vi "Generate Trajectory.vi"(8 "Conditions":T2, 9 "Limits":T1={"Velocity (fps)"=6.0, "Acceleration (fps^2)"=15.0, "Jerk (fps^3)"=100.0}, 10 "WayPoints":cluster{"x":dbl, "y":dbl, "th":dbl}[](array[cluster]), 11 "Sample Period (s)":dbl=0.02) -> (0 "Updated Waypoints":cluster{"x":dbl, "y":dbl, "th":dbl}[](array[cluster]), 1 "Valid":bool, 2 "Time (s)":dbl, 3 "Trajectory Data":T3(array[cluster]), 4 "Distance (ft)":dbl)   [LabVIEW 2018]
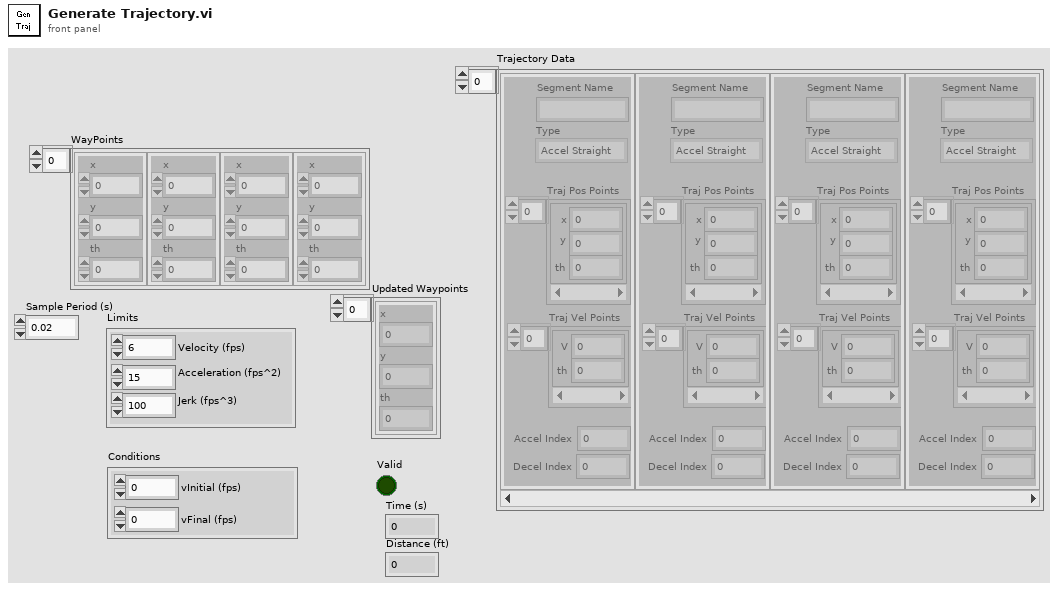
[diagram p1: front panel]
types:
  T1 = cluster{"Velocity (fps)":dbl, "Acceleration (fps^2)":dbl, "Jerk (fps^3)":dbl}
  T2 = cluster{"vInitial (fps)":dbl, "vFinal (fps)":dbl}
  T3 = cluster{"Segment Name":string, "Type":enum16{"Accel Straight", "Const Straight", "Blend", "Circle"}, "Traj Pos Points":cluster{"x":dbl, "y":dbl, "th":dbl}[], "Traj Vel Points":cluster{"V":dbl, "th":dbl}[], "Accel Index":i32, "Decel Index":i32}[]
  T4 = cluster{"distance (ft)":dbl, "dist of baseline Jerk":dbl, "dist of high Jerk":dbl}
  T5 = cluster{"Velocity (fps)":dbl, "Acceleration (fps^2)":dbl, "vInitial (fps)":dbl, "Sample Period (s)":dbl, "Jerk (fps^3)":dbl, cluster{"distance (ft)":dbl, "dist of baseline Jerk":dbl, "dist of high Jerk":dbl}, cluster{"distance (ft)":dbl, "dist of baseline Jerk":dbl, "dist of high Jerk":dbl}}
  T6 = cluster{"Point Out":cluster{"x":dbl, "y":dbl, "th":dbl}, "Point Out":cluster{"x":dbl, "y":dbl, "th":dbl}, "Valid":bool}[]
  T7 = typedef "BlendType.ctl" = cluster{"Scaling":dbl, "Length":dbl, "Angle":dbl, "Vertex Dist":dbl, "ParaTime":dbl, "ExtraArc":dbl, "Center Point":cluster{dbl, dbl}}
  T8 = cluster{"Velocity (fps)":dbl, "Velocity (fps)":dbl}
  T9 = cluster{"Segment Name":string, "Type":enum16{"Accel Straight", "Const Straight", "Blend", "Circle"}, "Traj Pos Points":cluster{"x":dbl, "y":dbl, "th":dbl}[], "Traj Vel Points":cluster{"V":dbl, "th":dbl}[], "Accel Index":i32, "Decel Index":i32}
  T10 = cluster{"maxV (fps)":dbl, "Accel Limit (fps^2)":dbl, "Initial V (fps)":dbl, "Sample Period (s)":dbl, "Jerk Limit (fps^3)":dbl, "Front Distances":cluster{"distance (ft)":dbl, "baseline (ft)":dbl, "high (ft)":dbl}, "Back Distances":cluster{"distance (ft)":dbl, "baseline (ft)":dbl, "high (ft)":dbl}}
  T11 = cluster{"maxV (fps)":dbl, "Accel Limit (fps^2)":dbl, "Initial V (fps)":dbl, "Sample Period (s)":dbl, "Jerk Limit (fps^3)":dbl, "Jerk Distances":cluster{"distance (ft)":dbl, dbl, dbl}, "Jerk Distances":cluster{"distance (ft)":dbl, dbl, dbl}}
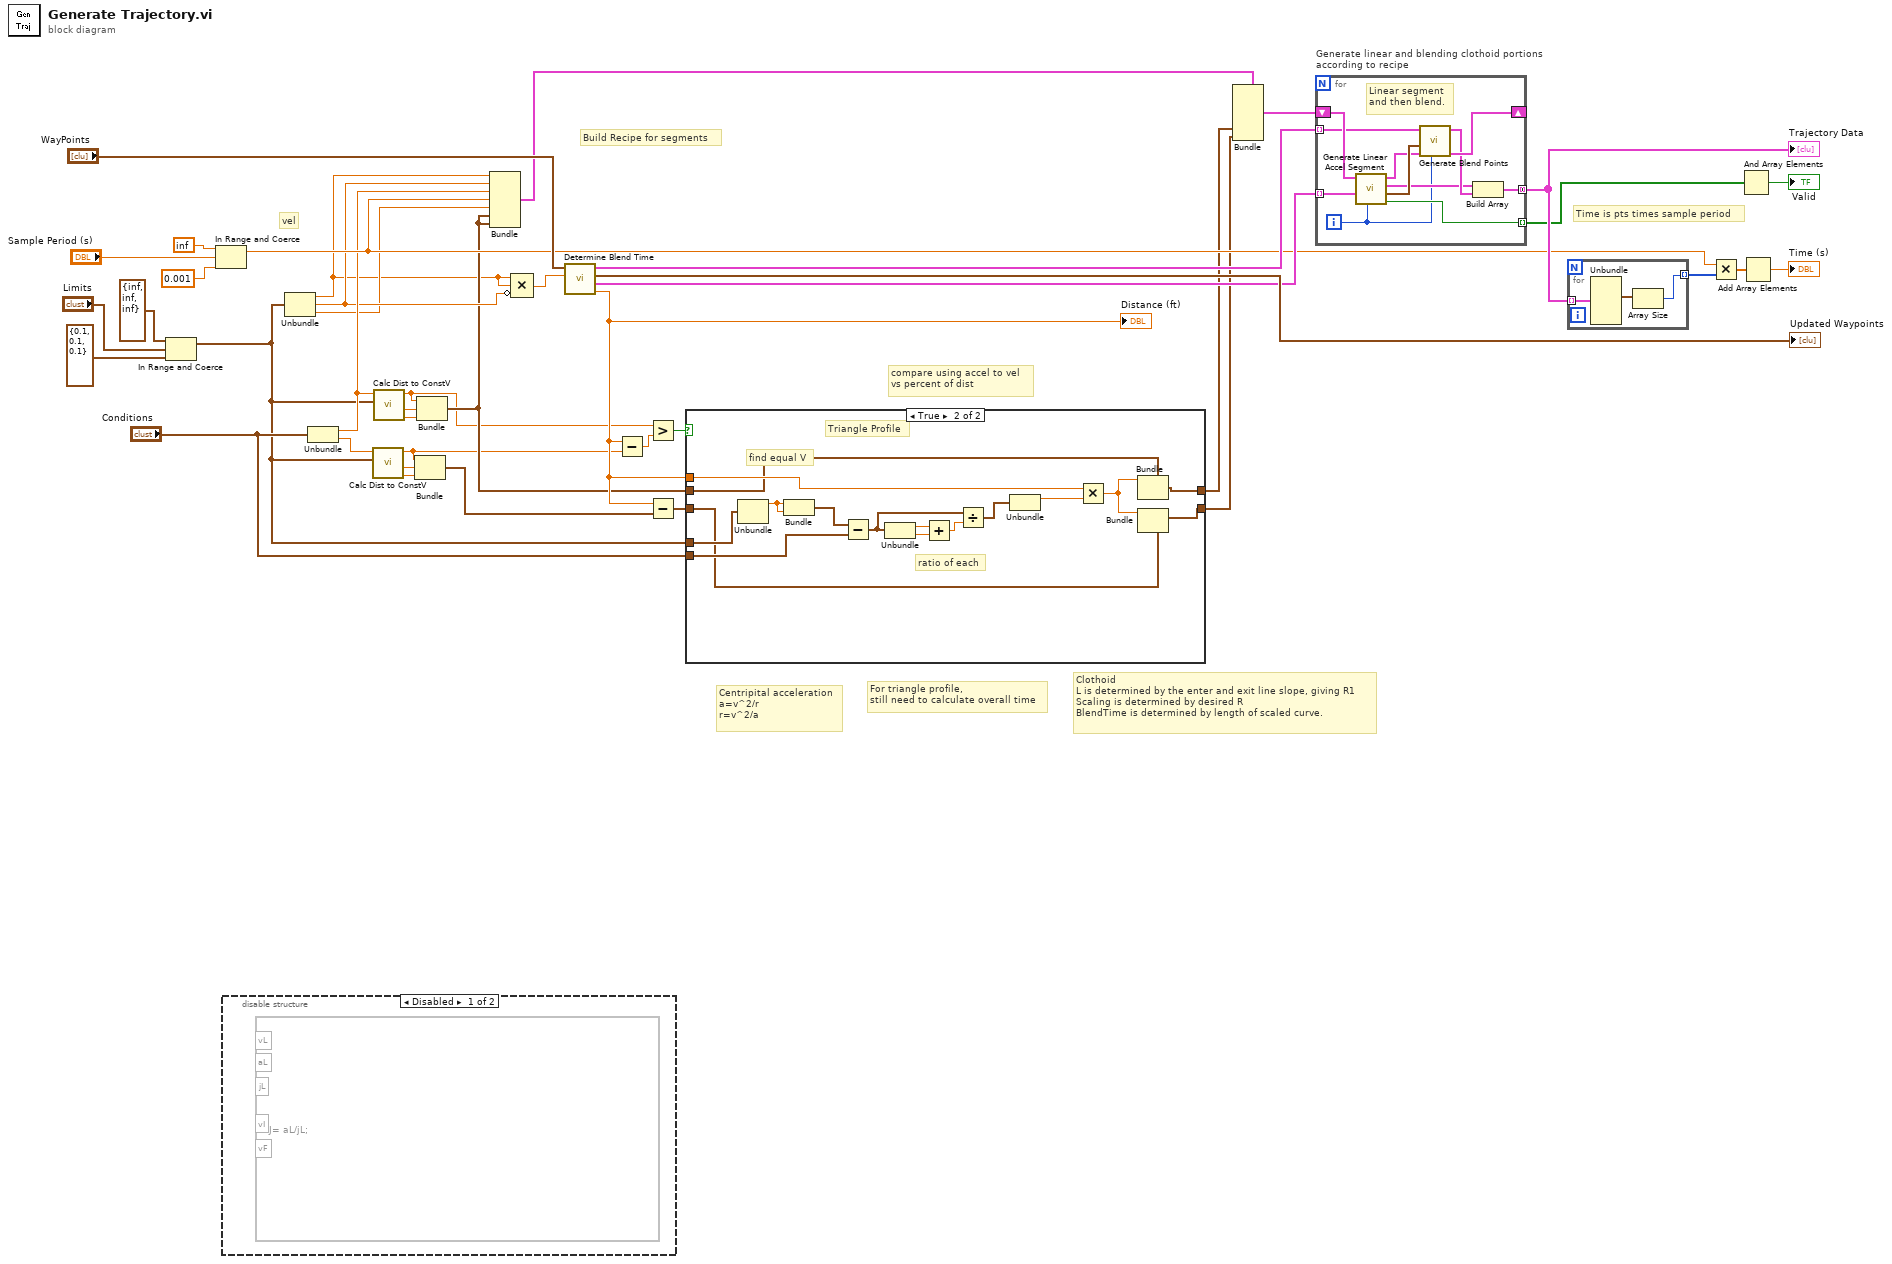
[diagram p0: block diagram]
diagram:
  # "For triangle profile,\nstill need to calculate overall time"
  # "compare using accel to vel\nvs percent of dist"
  # "Build Recipe for segments"
  # "Time is pts times sample period"
  # "Clothoid\nL is determined by the enter and exit line slope, giving R1\nScaling is determined by desired R\nBlendTime is determined by length of scaled curve."
  # "Centripital acceleration\na=v^2/r\nr=v^2/a"
  # "vel"
  n1 = In Range and Coerce(upper limit=T1 {"Velocity (fps)"=inf, "Acceleration (fps^2)"=inf, "Jerk (fps^3)"=inf}, x="Limits", lower limit=T1 {"Velocity (fps)"=0.1, "Acceleration (fps^2)"=0.1, "Jerk (fps^3)"=0.1} ("upper limit")) -> (coerced(x)=w14:T1)  [unwired: 1 out]
  n2 = In Range and Coerce(upper limit=inf, x="Sample Period (s)", lower limit=0.001) -> (coerced(x)=w25:dbl)  [unwired: 1 out]
  n3 = disable-structure shown="Disabled" {
    frame Disabled {
      n4 = formula code="tJ= aL/jL;"() -> ()  [unwired: 5 in]
    }
    frame Enabled {
    }
  }
  n5 = Unbundle(w14) -> ("Velocity (fps)"=w1:dbl, "Acceleration (fps^2)"=w16:dbl, "Jerk (fps^3)"=w15:dbl)
  n6 = Unbundle("Conditions") -> ("vInitial (fps)"=w21:dbl, "vFinal (fps)"=w20:dbl)
  n7 = call "Calc Dist to ConstV.vi"("Limits"=w14, "V endpoint (fps)"=w20) -> ("dist of high Jerk"=w11:dbl, "dist of baseline Jerk"=w10:dbl, "distance (ft)"=w4:dbl)  [unwired: 6 in, 1 out]
  n8 = call "Calc Dist to ConstV.vi"("Limits"=w14, "V endpoint (fps)"=w21) -> ("dist of high Jerk"=w13:dbl, "dist of baseline Jerk"=w12:dbl, "distance (ft)"=w5:dbl)  [unwired: 6 in, 1 out]
  n9 = Bundle("distance (ft)"=w4, "dist of baseline Jerk"=w10, "dist of high Jerk"=w11) -> (w8:T4)  [unwired: 1 in]
  n10 = Bundle("distance (ft)"=w5, "dist of baseline Jerk"=w12, "dist of high Jerk"=w13) -> (w6:T4)  [unwired: 1 in]
  n11 = Bundle("Velocity (fps)"=w1, "Acceleration (fps^2)"=w16, "vInitial (fps)"=w21, "Sample Period (s)"=w25, "Jerk (fps^3)"=w15, w6, w6) -> (w27:T5)  [unwired: 1 in]
  n12 = Compound Arithmetic op=MULTIPLY(w1, w1, invert w16) -> (w39:dbl)
  n13 = call "Determine Blend Time.vi"("Min R"=w39, "WayPoints"="WayPoints") -> ("Distance"=w9:dbl, "Linear Info"=w36:T6, "Updated Waypoints"=→"Updated Waypoints":cluster{"x":dbl, "y":dbl, "th":dbl}[], "Blends"=w35:T7[])  [unwired: 6 in]
  "Distance (ft)" <- w9
  n14 = Subtract(x=w9, y=w4) -> (x-y=w17:dbl)
  n15 = Greater?(x=w5, y=w17) -> (0:w19:bool)
  n16 = Subtract(x=w9, y=w8) -> (x-y=w7:T4)
  n17 = case shown="True" w19 {
    tunnel: w14 -> [_ w59]
    tunnel: "Conditions" -> [_ w56]
    tunnel: w9 -> [_ w46]
    tunnel: w6 -> [w43 w45]
    tunnel: [w43 w49] -> w3
    tunnel: w7 -> [w42 w44]
    tunnel: [w42 w48] -> w2
    frame False {
      # "Trapezoid Profile"
    }
    frame True {
      # "Triangle Profile"
      # "ratio of each"
      # "find equal V"
      n18 = Unbundle(w59) -> ("Velocity (fps)"=w58:dbl)  [unwired: 2 out]
      n19 = Bundle("Velocity (fps)"=w58, "Velocity (fps)"=w58) -> (w57:T8)  [unwired: 1 in]
      n20 = Subtract(x=w57, y=w56) -> (x-y=w53:cluster{dbl, dbl})
      n21 = Unbundle(w53) -> (w55:dbl, w54:dbl)
      n22 = Add(x=w55, y=w54) -> (x+y=w52:dbl)
      n23 = Divide(x=w53, y=w52) -> (x/y=w51:cluster{dbl, dbl})
      n24 = Unbundle(w51) -> (w50:dbl)  [unwired: 1 out]
      n25 = Multiply(x=w46, y=w50) -> (x*y=w47:dbl)
      n26 = Bundle(cluster=w45, "distance (ft)"=w47) -> (w49:T4)  [unwired: 2 in]
      n27 = Bundle(cluster=w44, "distance (ft)"=w47) -> (w48:T4)  [unwired: 2 in]
    }
  }
  n28 = Bundle(cluster=w27, w3, w2) -> (w26:T5)  [unwired: 5 in]
  n29 = for "Generate linear and blending clothoid portions\naccording to recipe" {
    tunnel: [w70] -> w32 mode=concatenating
    tunnel: w35 -> [w62] mode=indexing
    shift-right: [w69] -> _
    shift-left: w26 -> [w68]
    tunnel: w36 -> [w63] mode=indexing
    tunnel: [w61] -> w30 mode=indexing
    i -> [w60]
    # "Linear segment\nand then blend."
    n30 = call "Generate Linear Accel Segment.vi"("Index"=w60, "Linear Info"=w63, "Speeds"=w68) -> ("Valid"=w61:bool, "Final Position"=w67:cluster{dbl, dbl, dbl}, "Trajectory Segment"=w65:T9, "Speeds Out"=w64:T10)  [unwired: 5 in]
    n31 = call "Generate Blend Points.vi"("Index"=w60, "Speeds"=w64, "Initial Point"=w67, "Blend Info"=w62) -> ("Speeds Out"=w69:T11, "Trajectory Segment"=w66:T9)  [unwired: 6 in]
    n32 = Build Array(w65, w66) -> (w70:T3)
  }
  "Trajectory Data" <- w32
  n33 = for {
    tunnel: w32 -> [w73] mode=indexing
    tunnel: [w72] -> w34 mode=indexing
    n34 = Unbundle(w73) -> ("Traj Pos Points"=w71:cluster{"x":dbl, "y":dbl, "th":dbl}[])  [unwired: 5 out]
    n35 = Array Size(array=w71) -> (size(s)=w72:i32)
  }
  n36 = Multiply(x=w25, y=w34) -> (x*y=w33:dbl[])
  n37 = And Array Elements(Boolean array=w30) -> (logical AND=→"Valid":bool)
  n38 = Add Array Elements(numeric array=w33) -> (sum=→"Time (s)":dbl)
